vi "GetType.vi"(8 "error in (no error)":errorcluster, 11 "Clear Arbitrary Waveform [ARB] Msg":refnum<class "Clear Arbitrary Waveform [ARB] Msg.lvclass">) -> (0 "error out":errorcluster, 2 "Data Sample":variant, 3 "Clear Arbitrary Waveform [ARB] Msg":refnum<class "Clear Arbitrary Waveform [ARB] Msg.lvclass">)   [LabVIEW 2016, in "CS++Fgen.lvlib" / "Clear Arbitrary Waveform [ARB] Msg.lvclass"]
doc: "This VI delivers a sample of the data type format the message expects."
uses:
  Clear Arbitrary Waveform [ARB] Msg.lvclass
  Clear Arbitrary Waveform [ARB] Msg.lvclass/Clear Arbitrary Waveform [ARB] Msg.ctl
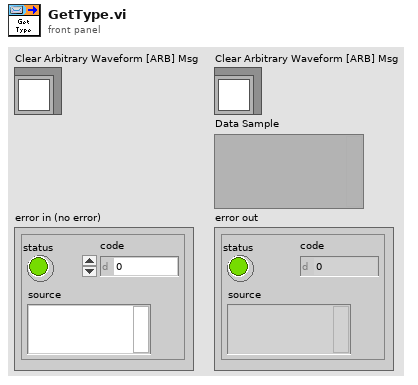
[diagram p1: front panel]
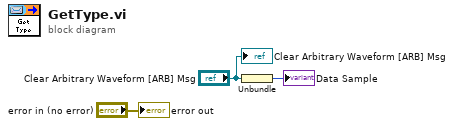
[diagram p0: block diagram]
diagram:
  n1 = Unbundle("Clear Arbitrary Waveform [ARB] Msg") -> (→"Data Sample":i32)
  "error out" <- "error in (no error)"
  "Clear Arbitrary Waveform [ARB] Msg" <- "Clear Arbitrary Waveform [ARB] Msg"
